vi "SVT UFF58 Read Record 4.vi"(0 "function refnum":refnum<k20>, 11 "error in (no error)":errorcluster) -> (4 "dup function refnum":refnum<k20>, 6 "record 4":string, 15 "error out":errorcluster)   [LabVIEW 2017, in "SoundVib_UFF58.lvlib"]
doc: "Reads the values of all the fields in record 4 of a UFF58 (universal file format) file."
uses:
  <vilib>/addons/Sound and Vibration/svt_UFF58/SoundVib_UFF58.lvlib
  <vilib>/Platform/storage/Storage.llb/Get Property (String).vi
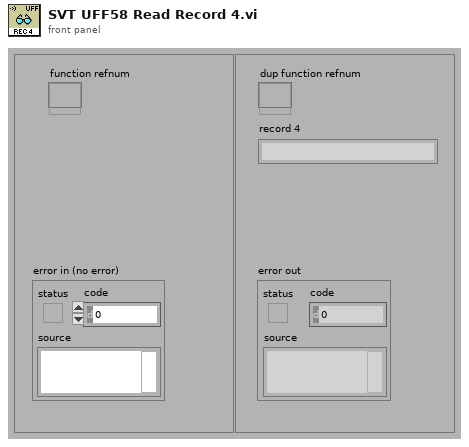
[diagram p1: front panel]
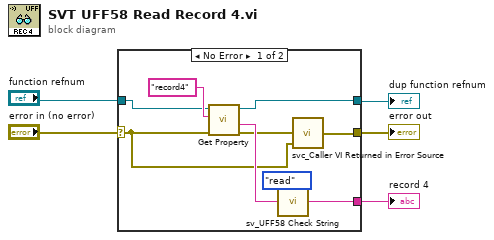
[diagram p0: block diagram]
diagram:
  n1 = case shown="No Error" "error in (no error)" {
    selector: "error in (no error)" -> [w6 w15]
    tunnel: "function refnum" -> [w7 w16]
    tunnel: [w10 w16] -> w2
    tunnel: [w13 w15] -> w5
    tunnel: [w9 _] -> w1
    frame No Error {
      n2 = call-poly <vilib>:"Get Property.vi"("error in (no error)"=w6, "Property name"="record4", "storage refnum"=w7) -> ("error out"=w11:errorcluster, "Value"=w12:string, "storage refnum out"=w10:refnum<k20>)  [unwired: 6 in]
      n3 = call <vilib>:"sv_UFF58 Check String.vi"("operation"=enum16{"read", "write"}."read", "field value"=w12) -> ("output string"=w9:string)  [unwired: 12 in, 1 out]
      n4 = call <vilib>:"svc_Caller VI Returned in Error Source.vi"("warning input to caller"=w6, "error in (no error)"=w11) -> ("error out"=w13:errorcluster)  [unwired: 3 in]
    }
    frame Error {
    }
  }
  "error out" <- w5
  "dup function refnum" <- w2
  "record 4" <- w1
